vi "clear_conversation_history.vi"(8 "error in (no error)":errorcluster, 11 "agent_simple_qa in":refnum<class "agent_simple_qa.lvclass">) -> (0 "error out":errorcluster, 3 "agent_simple_qa out":refnum<class "agent_simple_qa.lvclass">)   [LabVIEW 2020, in "agent_simple_qa.lvclass"]
uses:
  agent_simple_qa.lvclass
  models/abstract_message_base/abstract_message_base.lvclass
  agent_simple_qa.lvclass/agent_simple_qa.ctl
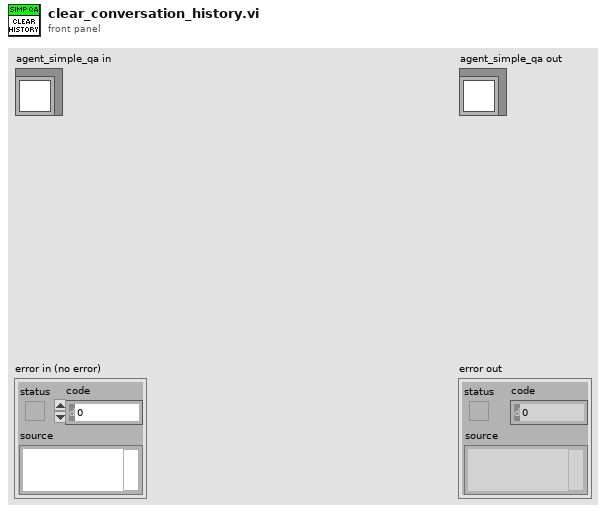
[diagram p1: front panel]
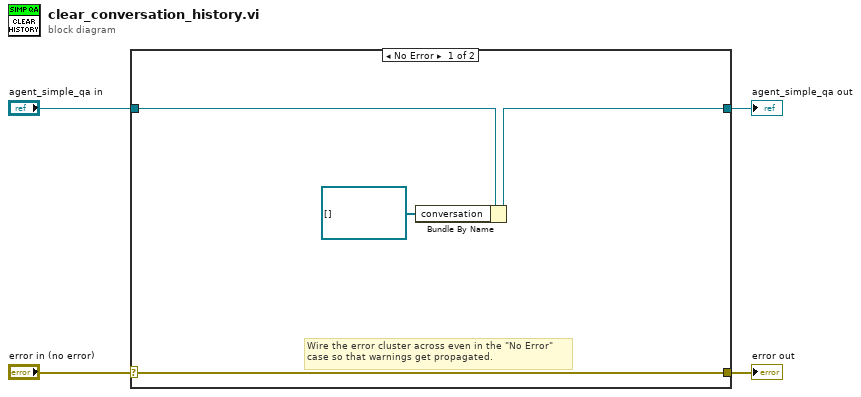
[diagram p0: block diagram]
diagram:
  n1 = case shown="No Error" "error in (no error)" {
    selector: "error in (no error)" -> [w8 w10]
    tunnel: [w8 w10] -> w3
    tunnel: [w7 w9] -> w1
    tunnel: "agent_simple_qa in" -> [w6 w9]
    frame No Error {
      # "Wire the error cluster across even in the \"No Error\"\ncase so that warnings get propagated."
      n2 = Bundle By Name(cluster=w6, "conversation"=refnum<class "abstract_message_base.lvclass">[] []) -> (w7:refnum<class "agent_simple_qa.lvclass">)
    }
    frame Error {
    }
  }
  "error out" <- w3
  "agent_simple_qa out" <- w1
